vi "应用程序各类属性.vi"() -> ()   [LabVIEW 2011]
panel:
  out "Application:User Name":string
  out "Application:Language":string
  out "Application:Directory Path":path
  out "Application:Name":string
  out "Application:Version Number":string
  out "Operating System:Name":string
  out "Operating System:Version Number":string
  out "Printing:Default Printer":string
  out "Printing:Available Printers":string[](array[string])
  out "bottom":i16
  out "resulting string":string
  out "x = y?":bool
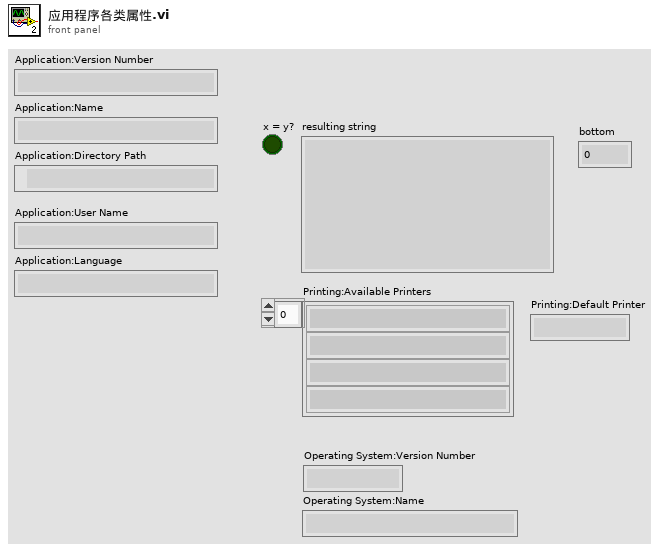
[diagram p1: front panel]
types:
  T1 = typedef "LVAllMonitorsDisplayTypeDef.ctl" = cluster{"Bounds":cluster{"Left":i16, "Top":i16, "Right":i16, "Bottom":i16}, "Depth":i16}[]
  T2 = typedef "LVRectTypeDef.ctl" = cluster{"left":i16, "top":i16, "right":i16, "bottom":i16}
  T3 = cluster{"Bounds":cluster{"Left":i16, "Top":i16, "Right":i16, "Bottom":i16}, "Depth":i16}
  T4 = cluster{"Left":i16, "Top":i16, "Right":i16, "Bottom":i16}
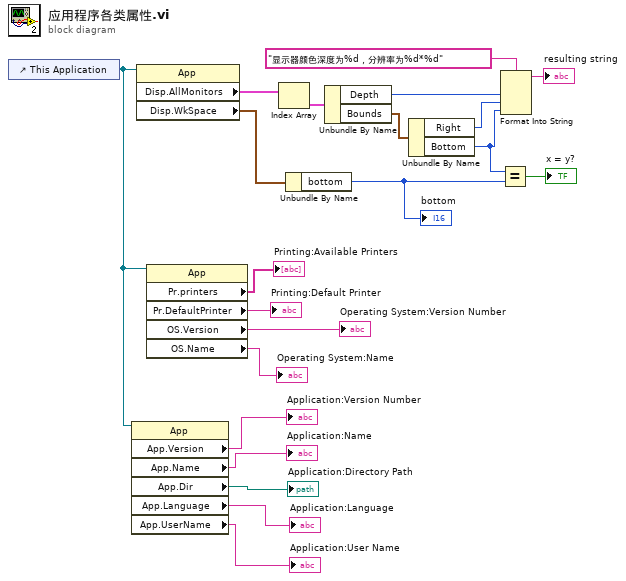
[diagram p0: block diagram]
diagram:
  n1 = control-ref of="This Application"() -> (w6:refnum<vi>)
  n2 = property class="App"(reference=w6) -> ("App.Version"=→"Application:Version Number":string, "App.Name"=→"Application:Name":string, "App.Dir"=→"Application:Directory Path":path, "App.Language"=→"Application:Language":string, "App.UserName"=→"Application:User Name":string)  [unwired: 1 in, 2 out]
  n3 = property class="App"(reference=w6) -> ("Disp.AllMonitors"=w21:T1, "Disp.WkSpace"=w19:T2)  [unwired: 1 in, 2 out]
  n4 = property class="App"(reference=w6) -> ("Pr.printers"=→"Printing:Available Printers":string[], "Pr.DefaultPrinter"=→"Printing:Default Printer":string, "OS.Version"=→"Operating System:Version Number":string, "OS.Name"=→"Operating System:Name":string)  [unwired: 1 in, 2 out]
  n5 = Index Array(array=w21) -> (element=w20:T3)  [unwired: 1 in]
  n6 = Unbundle By Name(w19) -> ("bottom"=w13:i16)
  "bottom" <- w13
  n7 = Unbundle By Name(w20) -> ("Depth"=w16:i16, "Bounds"=w18:T4)
  n8 = Unbundle By Name(w18) -> ("Right"=w15:i16, "Bottom"=w14:i16)
  n9 = Equal?(x=w14, y=w13) -> (x = y?=→"x = y?":bool)
  n10 = Format Into String(format string="显示器颜色深度为%d，分辨率为%d*%d", w16, w15, w14) -> (resulting string=→"resulting string":string)  [unwired: 2 in, 1 out]
